vi "Dashboard Main.vi"() -> ()   [LabVIEW 2011]
uses:
  <vilib>/Rock Robotics/WPI/Camera/WPI_CameraImageSize.ctl
  <vilib>/Rock Robotics/WPI/DriverStation/WPI_DriverStationDigitalData.ctl
  <vilib>/Rock Robotics/WPI/Camera/WPI_CameraWhite Balance Values.ctl
  <vilib>/vision/NI_Vision_Development_Module.lvlib
panel:
  out "fps":dbl
  in  "Miliseconds":u32=500
  in  "Camera Settings":T2={"FPS"=10, "Compression"=30, "Image Size"=enum."320x240"}
  out "Processed Image":T3(plugin-control)
  out "Original Image":T3(plugin-control)
  in  "Annotate":bool=TRUE
  in  "Processing":enum32{"Color", "Intensity", "Intensity Open"}(tab)
  in  "Luminance":i32=255
  in  "Saturation":i32=255
  in  "Hue":i32(knob)=65 scale=0.0..255.0
  in  "Margins":cluster{"Hue":i32, "Sat":i32, "Lum":i32}={"Hue"=9, "Sat"=40, "Lum"=19} {"Sat" scale=0.0..40.0; "Lum" scale=0.0..40.0; "Hue" scale=0.0..40.0}
  in  "Range":cluster{"Lower value":sgl, "Upper value":sgl}={"Lower value"=150.0, "Upper value"=255.0} {"Lower value" scale=0.0..255.0; "Upper value" scale=0.0..255.0}
  in  "Range 2":cluster{"Lower value":sgl, "Upper value":sgl}={"Lower value"=150.0, "Upper value"=255.0} {"Lower value" scale=0.0..255.0; "Upper value" scale=0.0..255.0}
  out "Target Info":T4(array[cluster])
  in  "Particle Count Limit":i32=10
  in  "Area Size Limit":i32=444
  in  "Score Limits":T5={"Rect Coverage"=76.0, "Aspect Ratio"=70.0, "X Edge Strength"=40.0, "Y Edge Strength"=60.0}
  in  "Camera Type":enum16{"206", "1011"}(ring)
  in  "Viewer":enum32{"Camera Image", "Kinect Skeleton"}(tab)
  in  "Video Enable":bool=TRUE
  out "Camera Image":T3(plugin-control)
  out "Buttons 1":cluster{"1":bool, "2":bool, "3":bool}
  out "Kinect 1":cluster{"X":dbl, "Y":dbl, "Z":dbl} {"X" scale=1.0..-1.0; "Y" scale=1.0..-1.0; "Z" scale=1.0..-1.0}
  out "Buttons 2":cluster{"1":bool, "2":bool, "3":bool}
  out "Kinect 2":cluster{"X":dbl, "Y":dbl, "Z":dbl} {"X" scale=1.0..-1.0; "Y" scale=1.0..-1.0; "Z" scale=1.0..-1.0}
  out "Version":string
  out "Skeleton Picture":picture
  out "Players":i8
  out "Dashboard Datatype Warning":string="Warning: The Dashboard Datatype used by the robot project and this dashboard do not match.\nSee diagram for more details."
  out "Robot IP Address":string
  out "Image Error Message":string="Timeout in Camera Communications"
  # "Communications"
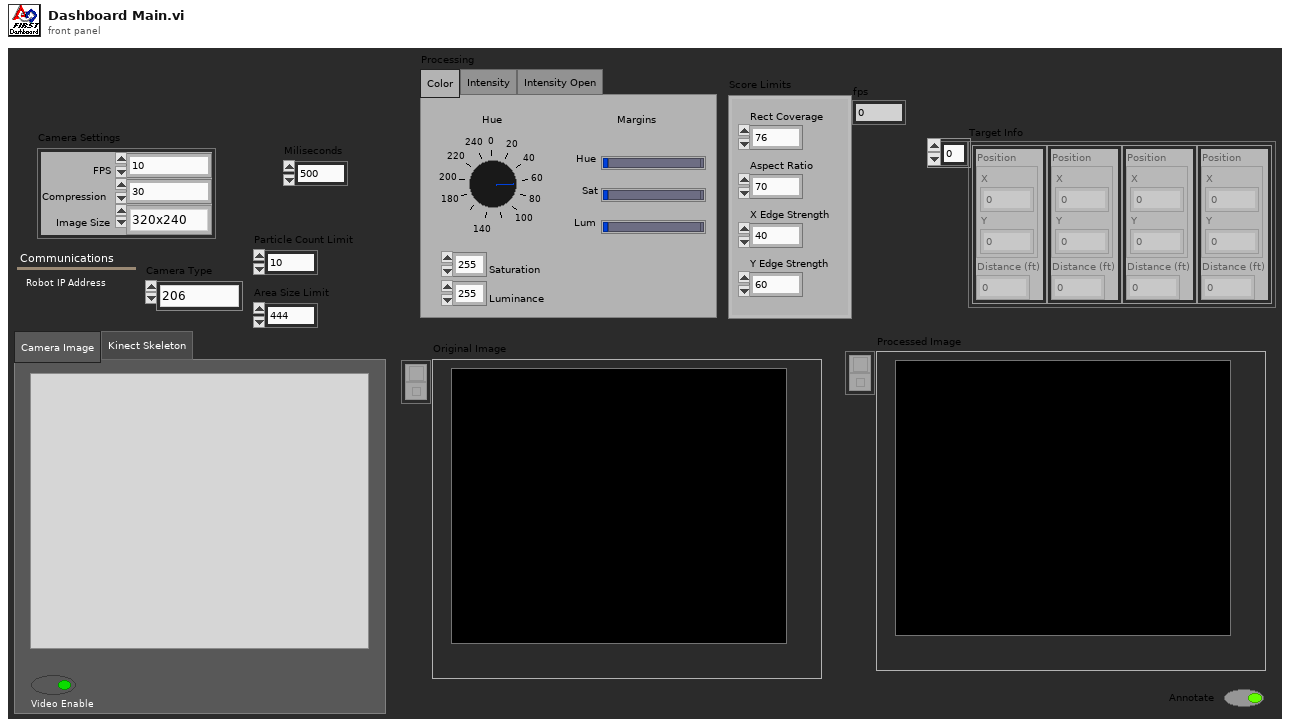
[diagram p1: front panel]
types:
  T1 = typedef "WPI_CameraImageSize.ctl" = enum16{"640x480", "320x240", "160x120"}
  T2 = cluster{"FPS":i32, "Compression":i32, "Image Size":T1}
  T3 = typedef "IMAQ Image.ctl" = refnum<image>
  T4 = cluster{"Position":cluster{"X":dbl, "Y":dbl}, "Distance (ft)":dbl}[]
  T5 = cluster{"Rect Coverage":dbl, "Aspect Ratio":dbl, "X Edge Strength":dbl, "Y Edge Strength":dbl}
  T6 = typedef "WPI_CameraWhite Balance Values.ctl" = enum16{"Auto", "Fixed indoor", "Fixed outdoor 1", "Fixed outdoor 2", "Fixed fluorescent 1", "Fixed fluorescent 2", "Hold current"}
  T7 = typedef "Image Type" = u32
  T8 = typedef "WPI_DriverStationDigitalData.ctl" = cluster{"Relay Fwd":u8, "Relay Rev":u8, "GPIO":u16, "GPIO_OE":u16, "PWM":cluster{"PWM[0]":u8, "PWM[1]":u8, "PWM[2]":u8, "PWM[3]":u8, "PWM[4]":u8, "PWM[5]":u8, "PWM[6]":u8, "PWM[7]":u8, "PWM[8]":u8, "PWM[9]":u8}}
  T9 = cluster{cluster{"AnalogModule[0]":cluster{"Channel[0]":sgl, "Channel[1]":sgl, "Channel[2]":sgl, "Channel[3]":sgl, "Channel[4]":sgl, "Channel[5]":sgl, "Channel[6]":sgl, "Channel[7]":sgl}, "AnalogModule[1]":cluster{"Channel[0]":sgl, "Channel[1]":sgl, "Channel[2]":sgl, "Channel[3]":sgl, "Channel[4]":sgl, "Channel[5]":sgl, "Channel[6]":sgl, "Channel[7]":sgl}}, cluster{"DigitalModule[0]":T8, "DigitalModule[1]":T8}, "Solenoid":u8}
  T10 = typedef "WPI_CameraDevRef.ctl" = cluster{"Camera Address":string, "CameraStatus":errorcluster, "Acquire Image Notifier":refnum<notifier>}
  T11 = typedef "LVBoundsTypeDef.ctl" = cluster{"Width":u32, "Height":u32}
  T12 = typedef "SkeletonTrackState.ctl" = enum32{"NotTracked", "PositionOnly", "Tracked"}
  T13 = cluster{"TrackingState":u8[], "Position":cluster{"x":sgl, "y":sgl, "z":sgl}, cluster{"x":sgl, "y":sgl, "z":sgl, sgl}[], "TrackState":T12}
  T14 = cluster{cluster{"ScaledToPercentRange":dbl, "ScaledToPercentRange":dbl, "ScaledToPercentRange":dbl}, cluster{bool, bool, bool}}[]
  T15 = cluster{cluster{"ScaledToPercentRange":dbl, "ScaledToPercentRange":dbl, "ScaledToPercentRange":dbl}, cluster{bool, bool, bool}}
  T16 = cluster{"ScaledToPercentRange":dbl, "ScaledToPercentRange":dbl, "ScaledToPercentRange":dbl}
  T17 = cluster{"Competition mode":bool, "Robot Link":bool, "Autonomous":bool, "Enabled":bool, "E-Stop":bool}
  T18 = cluster{"AnalogModule[0]":cluster{"Channel[0]":sgl, "Channel[1]":sgl, "Channel[2]":sgl, "Channel[3]":sgl, "Channel[4]":sgl, "Channel[5]":sgl, "Channel[6]":sgl, "Channel[7]":sgl}, "AnalogModule[1]":cluster{"Channel[0]":sgl, "Channel[1]":sgl, "Channel[2]":sgl, "Channel[3]":sgl, "Channel[4]":sgl, "Channel[5]":sgl, "Channel[6]":sgl, "Channel[7]":sgl}}
  T19 = cluster{"DigitalModule[0]":T8, "DigitalModule[1]":T8}
  T20 = cluster{"Channel[0]":sgl, "Channel[1]":sgl, "Channel[2]":sgl, "Channel[3]":sgl, "Channel[4]":sgl, "Channel[5]":sgl, "Channel[6]":sgl, "Channel[7]":sgl}[]
  T21 = cluster{"Channel[0]":sgl, "Channel[1]":sgl, "Channel[2]":sgl, "Channel[3]":sgl, "Channel[4]":sgl, "Channel[5]":sgl, "Channel[6]":sgl, "Channel[7]":sgl}
  T22 = typedef "LVRectTypeDef.ctl" = cluster{"left":i16, "top":i16, "right":i16, "bottom":i16}
  T23 = cluster{"Left":dbl, "Top":dbl, "Right":dbl, "Bottom":dbl}
  T24 = enum32{"AutoM", "Close", "Dilate", "Erode", "Gradient", "Gradient out", "Gradient in", "Hit miss", "Open", "PClose", "POpen", "Thick", "Thin"}
  T25 = cluster{cluster{"Left":dbl, "Top":dbl, "Right":dbl, "Bottom":dbl}, dbl[]}[]
  T26 = cluster{"Target Center (-1 to 1)":cluster{"X":dbl, "Y":dbl}, "Distance (ft)":dbl}
  T27 = cluster{"Target Center (-1 to 1)":cluster{"X":dbl, "Y":dbl}, "Distance (ft)":dbl}[]
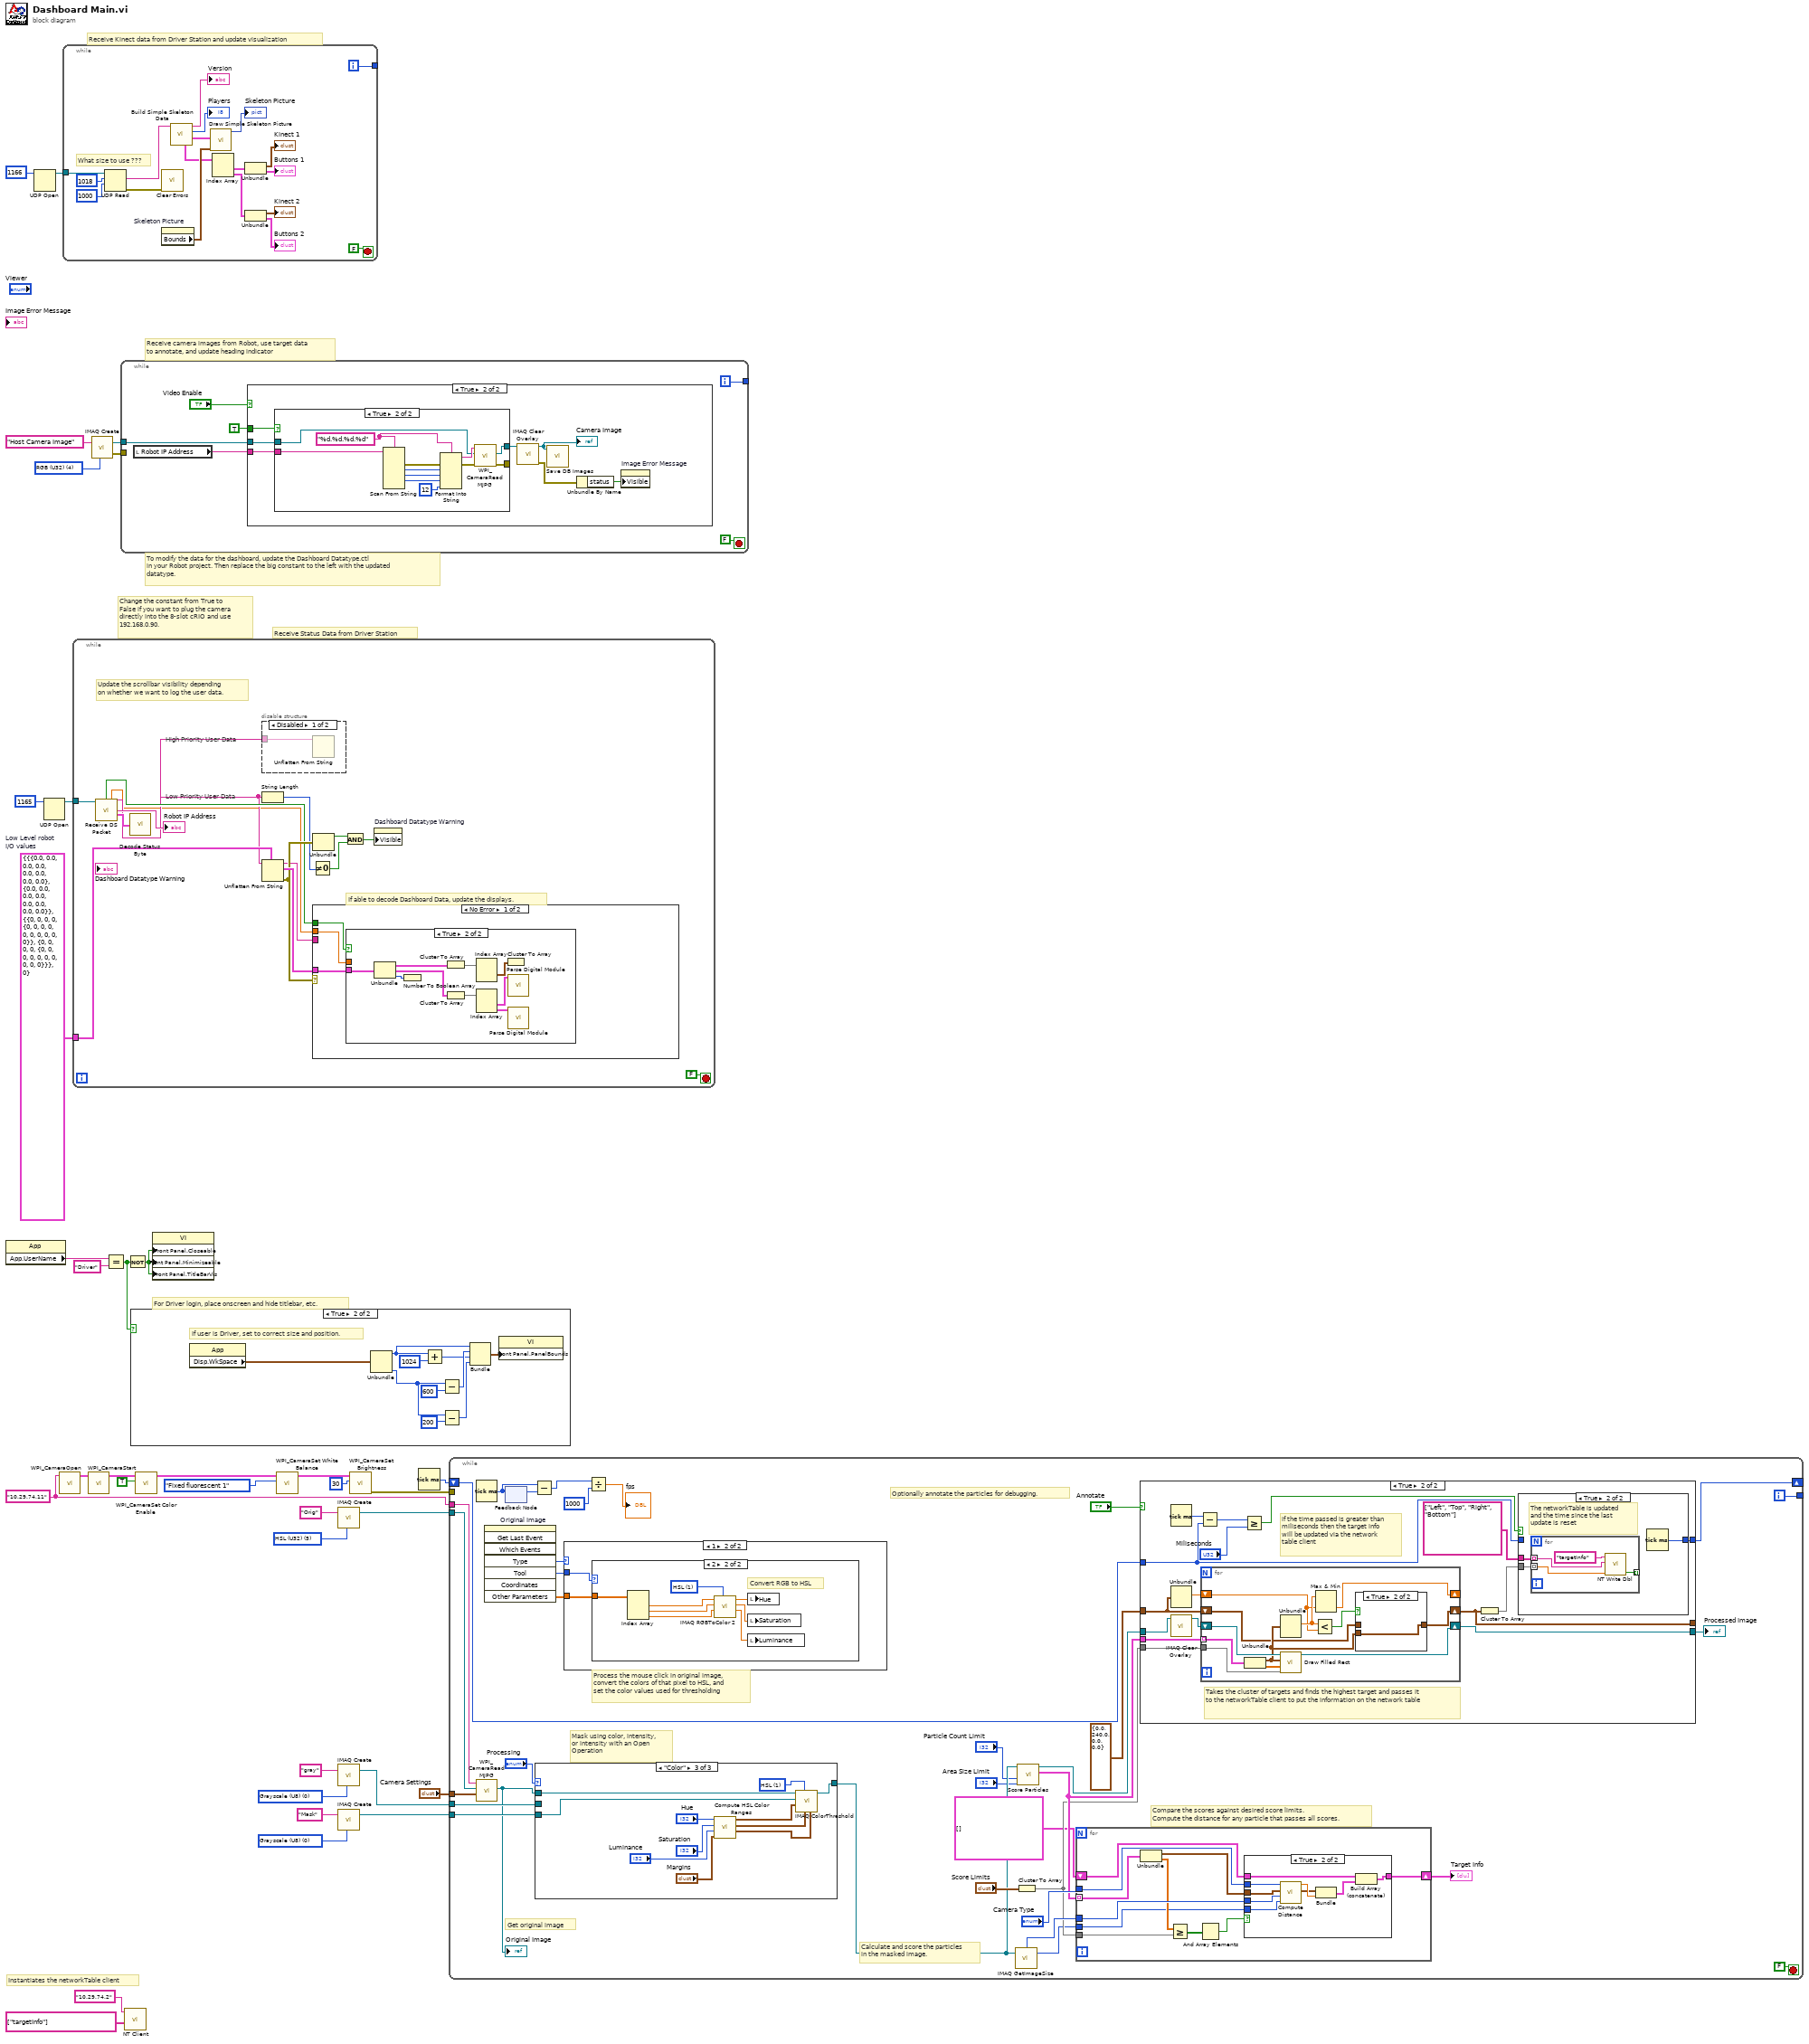
[diagram p0: block diagram]
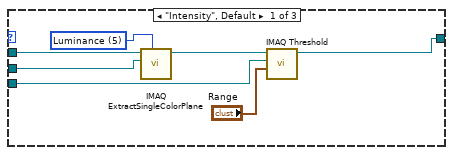
[diagram p5: hidden frame]
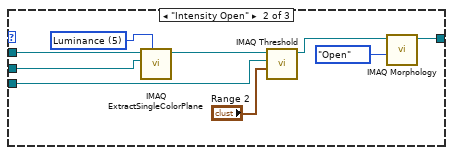
[diagram p6: hidden frame]
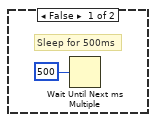
[diagram p14: hidden frame]
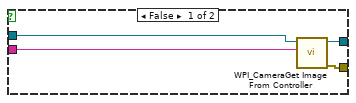
[diagram p15: hidden frame]
diagram:
  w1 = "10.29.74.11" ("Camera IP Address")
  w15 = T7 0 items=["Grayscale (U8)", "Grayscale (I16)", "Grayscale (SGL)", "Complex (CSG)", "RGB (U32)", "HSL (U32)", "RGB (U64)", "Grayscale (U16)"] ("Image Type")
  w19 = T7 5 items=["Grayscale (U8)", "Grayscale (I16)", "Grayscale (SGL)", "Complex (CSG)", "RGB (U32)", "HSL (U32)", "RGB (U64)", "Grayscale (U16)"] ("Image Type")
  w22 = T7 0 items=["Grayscale (U8)", "Grayscale (I16)", "Grayscale (SGL)", "Complex (CSG)", "RGB (U32)", "HSL (U32)", "RGB (U64)", "Grayscale (U16)"] ("Image Type")
  w25 = T9 {{"AnalogModule[0]"={"Channel[0]"=0.0, "Channel[1]"=0.0, "Channel[2]"=0.0, "Channel[3]"=0.0, "Channel[4]"=0.0, "Channel[5]"=0.0, "Channel[6]"=0.0, "Channel[7]"=0.0}, "AnalogModule[1]"={"Channel[0]"=0.0, "Channel[1]"=0.0, "Channel[2]"=0.0, "Channel[3]"=0.0, "Channel[4]"=0.0, "Channel[5]"=0.0, "Channel[6]"=0.0, "Channel[7]"=0.0}}, {"DigitalModule[0]"={"Relay Fwd"=0, "Relay Rev"=0, "GPIO"=0, "GPIO_OE"=0, "PWM"={"PWM[0]"=0, "PWM[1]"=0, "PWM[2]"=0, "PWM[3]"=0, "PWM[4]"=0, "PWM[5]"=0, "PWM[6]"=0, "PWM[7]"=0, "PWM[8]"=0, "PWM[9]"=0}}, "DigitalModule[1]"={"Relay Fwd"=0, "Relay Rev"=0, "GPIO"=0, "GPIO_OE"=0, "PWM"={"PWM[0]"=0, "PWM[1]"=0, "PWM[2]"=0, "PWM[3]"=0, "PWM[4]"=0, "PWM[5]"=0, "PWM[6]"=0, "PWM[7]"=0, "PWM[8]"=0, "PWM[9]"=0}}}, "Solenoid"=0}  # Low Level robot I/O values
  w33 = T7 4 items=["Grayscale (U8)", "Grayscale (I16)", "Grayscale (SGL)", "Complex (CSG)", "RGB (U32)", "HSL (U32)", "RGB (U64)"] ("Image Type")
  # "Instantiates the networkTable client"
  # "Change the constant from True to\nFalse if you want to plug the camera\ndirectly into the 8-slot cRIO and use\n192.168.0.90."
  # "Receive Kinect data from Driver Station and update visualization"
  # "For Driver login, place onscreen and hide titlebar, etc."
  # "To modify the data for the dashboard, update the Dashboard Datatype.ctl\nin your Robot project. Then replace the big constant to the left with the updated\ndatatype."
  # "Receive Status Data from Driver Station"
  # "Receive camera images from Robot, use target data\nto annotate, and update heading indicator"
  n1 = property class="App"() -> ("App.UserName"=w28:string)  [unwired: 2 in, 2 out]
  n2 = UDP Open(11:u16 1166 ("port")) -> (port=w23:refnum<k16>)  [unwired: 2 in, 4 out]
  n3 = UDP Open(11:u16 1165 ("port")) -> (port=w34:refnum<k16>)  [unwired: 2 in, 4 out]
  n4 = call <vilib>:"WPI_CameraOpen.vi"("Camera Address"=w1) -> ("CameraDevRef"=w3:T10)  [unwired: 9 in, 1 out]
  n5 = while {
    tunnel: w23 -> [w52]
    tunnel: [w36] -> _
    i -> [w36]
    stop <- FALSE stop-if-true
    # "What size to use ???"
    n6 = UDP Read(connection ID=w52, max size (548)=1018 ("bytes to read"), timeout ms (25000)=1000) -> (data out=w46:string, error out=w44:errorcluster)  [unwired: 1 in, 3 out]
    n7 = call <vilib>:"Clear Errors.vi"("error in (no error)"=w44) -> ()  [unwired: 6 in, 1 out]
    n8 = property on="Skeleton Picture" class="Pict"() -> ("Bounds"=w48:T11)  [unwired: 2 in, 2 out]
    n9 = call "Build Simple Skeleton Data.vi"("data out"=w46) -> ("Skeleton Data"=w47:T13, "NumPlayers"=→"Players":i8, "Version String"=→"Version":string, "Simple Joystick Info"=w43:T14)  [unwired: 6 in, 1 out]
    n10 = call "Draw Simple Skeleton Picture.vi"("Bounds"=w48, "Simple Skeleton"=w47) -> ("new picture out"=→"Skeleton Picture":picture)  [unwired: 9 in]
    n11 = Index Array(array=w43) -> (element #1=w42:T15, element #2=w41:T15)  [unwired: 2 in]
    n12 = Unbundle(w42) -> (→"Kinect 1":T16, →"Buttons 1":cluster{bool, bool, bool})
    n13 = Unbundle(w41) -> (→"Kinect 2":T16, →"Buttons 2":cluster{bool, bool, bool})
  }
  n14 = while {
    tunnel: w34 -> [w68]
    tunnel: w25 -> [w67]
    stop <- FALSE stop-if-true
    # "High Priority User Data"
    # "Low Priority User Data"
    # "Update the scrollbar visibility depending\non whether we want to log the user data."
    # "If able to decode Dashboard Data, update the displays."
    n15 = call "Receive DS Packet.vi"("Recv Socket"=w68) -> ("New Dashboard Data"=w64:bool, "Battery"=w55:sgl, "Robot IP Address"=→"Robot IP Address":string, "Status"=w69:T17, "Low Priority User Data"=w57:string, "High Priority User Data"=w56:string)  [unwired: 1 in, 8 out]
    n16 = call "Decode Status Byte.vi"("Status Byte"=w69) -> ()  [unwired: 2 out]
    n17 = disable-structure shown="Disabled" {
      disable-tunnel: w56 -> [w71 _]
      frame Disabled {
        n18 = Unflatten From String(binary string=w71) -> ()  [unwired: 2 in, 5 out]
      }
      frame Enabled {
      }
    }
    n19 = String Length(string=w57) -> (length=w59:i32)
    n20 = Unflatten From String(type=w67, binary string=w57) -> (rest of the binary string=w60:string, value=w66:T9, error out=w65:errorcluster)  [unwired: 1 in, 2 out]
    n21 = Not Equal To 0?(x=w59) -> (x != 0?=w62:bool)
    n22 = Unbundle(w65) -> ("status"=w61:bool)  [unwired: 2 out]
    n23 = case shown="No Error" w65 {
      tunnel: w66 -> [w74 _]
      tunnel: w64 -> [w73 _]
      tunnel: w60 -> [_ _]
      tunnel: w55 -> [w72 _]
      frame No Error {
        n24 = case shown="True" w73 {
          tunnel: w74 -> [_ w79]
          tunnel: w72 -> [_ _]
          frame False {
            # "Don't update if the robot hasn't sent new data"
          }
          frame True {
            n25 = Unbundle(w79) -> (w76:T18, w77:T19, "Solenoid"=w78:u8)
            n26 = Number To Boolean Array(number=w78) -> ()  [unwired: 1 out]
            n27 = Cluster To Array(cluster=w76) -> (array=w83:T20)
            n28 = Cluster To Array(cluster=w77) -> (array=w82:T8[])
            n29 = Index Array(array=w83) -> (element #1=w75:T21)  [unwired: 2 in, 1 out]
            n30 = Index Array(array=w82) -> (element #1=w81:T8, element #2=w80:T8)  [unwired: 2 in]
            n31 = Cluster To Array(cluster=w75) -> ()  [unwired: 1 out]
            n32 = call "Parse Digital Module.vi"("DigitalModule"=w81) -> ()  [unwired: 11 out]
            n33 = call "Parse Digital Module.vi"("DigitalModule"=w80) -> ()  [unwired: 11 out]
          }
        }
      }
      frame Error {
        # "Your datatypes don't match. The Dashboard Datatype.ctl in your Robot project\nand the big constant to the left of the loop need to match."
      }
    }
    n34 = And(x=w61, y=w62) -> (x .and. y?=w63:bool)
    n35 = property on="Dashboard Datatype Warning" class="Str"("Visible"=w63) -> ()  [unwired: 2 in, 2 out]
  }
  n36 = call <vilib>:"WPI_CameraStart.vi"("CameraDevRef"=w3) -> ("CameraDevRef Out"=w2:T10)  [unwired: 9 in, 1 out]
  n37 = call "IMAQ Create"("Image Name"="Host Camera Image", "Image Type"=w33) -> ("New Image"=w31:T3, "error out"=w30:errorcluster)  [unwired: 2 in, 1 out]
  n38 = Equal?(x=w28, y="Driver") -> (x = y?=w27:bool)
  n39 = while {
    tunnel: w31 -> [w87]
    tunnel: w30 -> [_]
    tunnel: [w84] -> _
    i -> [w84]
    stop <- FALSE stop-if-true
    n40 = local read "Robot IP Address"() -> (w88:string)
    n41 = case shown="True" "Video Enable" {
      tunnel: w88 -> [_ w97]
      tunnel: w87 -> [_ w96]
      tunnel: TRUE -> [_ w91]
      frame False {
        # "Sleep for 500ms"
        n42 = Wait Until Next ms Multiple(millisecond multiple=u32 500) -> ()  [unwired: 1 out]
      }
      frame True {
        n43 = case shown="True" w91 {
          tunnel: w96 -> [w100 w107]
          tunnel: [w98 w105] -> _
          tunnel: [w99 w106] -> w93
          tunnel: w97 -> [w101 w110]
          frame False {
            n44 = call <vilib>:"WPI_CameraGet Image From Controller.vi"("Controller Address"=w101, "Image"=w100) -> ("error out"=w98:errorcluster, "Image Out"=w99:T3)  [unwired: 2 in, 6 out]
          }
          frame True {
            w102 = "%d.%d.%d.%d" ("format string")
            n45 = Scan From String(format string=w102, input string=w110) -> (error out=w109:errorcluster, output 1=w111:i32, output 2=w112:i32, output 3=w113:i32)  [unwired: 2 in, 7 out]
            n46 = Format Into String(format string=w102, error in=w109, w111, w112, w113, 12 ("IP Suffix:")) -> (resulting string=w108:string, error out=w104:errorcluster)  [unwired: 1 in]
            n47 = call <vilib>:"WPI_CameraRead MJPG.vi"("error in"=w104, "Image"=w107, "address"=w108) -> ("error out"=w105:errorcluster, "Image Out"=w106:T3)  [unwired: 7 in]
          }
        }
        n48 = call "IMAQ Clear Overlay"("Image"=w93) -> ("error out"=w94:errorcluster, "Image Out"=w92:T3)  [unwired: 2 in, 7 out]
        "Camera Image" <- w92
        n49 = call "Save DB Images.vi"("Image"=w92) -> ()  [unwired: 2 in, 1 out]
        n50 = Unbundle By Name(w94) -> ("status"=w95:bool)
        n51 = property on="Image Error Message" class="Str"("Visible"=w95) -> ()  [unwired: 2 in, 2 out]
      }
    }
  }
  n52 = call "NT Client.vi"("Requested Tables"=string[] ["targetInfo"], "server IP Address"="10.29.74.2") -> ()  [unwired: 10 in]
  n53 = Not(x=w27) -> (.not. x?=w26:bool)
  n54 = case shown="True" w27 {
    frame False {
    }
    frame True {
      # "If user is Driver, set to correct size and position."
      n55 = property class="App"() -> ("Disp.WkSpace"=w123:T22)  [unwired: 2 in, 2 out]
      n56 = Unbundle(w123) -> ("left"=w118:i16, "bottom"=w114:i16)  [unwired: 2 out]
      n57 = Add(x=w118, y=1024) -> (x+y=w119:i32)
      n58 = Subtract(x=w114, y=600) -> (x-y=w120:i32)
      n59 = Subtract(x=w114, y=200) -> (x-y=w115:i32)
      n60 = Bundle("left"=w118, w120, w119, w115) -> (w122:cluster{"left":i16, i32, i32, i32})  [unwired: 1 out]
      n61 = property class="VI"("Front Panel.PanelBounds"=w122) -> ()  [unwired: 2 in, 2 out]
    }
  }
  n62 = call <vilib>:"WPI_CameraSet Color Enable.vi"("Color Enabled"=TRUE, "CameraDevRef"=w2) -> ("CameraDevRef Out"=w12:T10)  [unwired: 8 in, 1 out]
  n63 = property class="VI"("Front Panel.Closeable"=w26, "Front Panel.Minimizeable"=w26, "Front Panel.TitleBarVis"=w26) -> ()  [unwired: 2 in, 2 out]
  n64 = call <vilib>:"WPI_CameraSet White Balance.vi"("White Balance"=WPI_CameraWhite_Balance_Values."Fixed fluorescent 1", "CameraDevRef"=w12) -> ("CameraDevRef Out"=w10:T10)  [unwired: 8 in, 1 out]
  n65 = call "IMAQ Create"("Image Name"="Orig", "Image Type"=w19) -> ("New Image"=w18:T3)  [unwired: 2 in, 2 out]
  n66 = call "IMAQ Create"("Image Name"="gray", "Image Type"=w22) -> ("New Image"=w17:T3)  [unwired: 2 in, 2 out]
  n67 = call "IMAQ Create"("Image Name"="Mask", "Image Type"=w15) -> ("New Image"=w14:T3)  [unwired: 2 in, 2 out]
  n68 = call <vilib>:"WPI_CameraSet Brightness.vi"("Brightness"=30, "CameraDevRef"=w10) -> ("error out"=w8:errorcluster)  [unwired: 8 in, 1 out]
  n69 = Tick Count (ms)() -> (millisecond timer value=w4:u32)
  n70 = while {
    tunnel: w18 -> [w129]
    tunnel: w17 -> [w157]
    tunnel: w14 -> [w156]
    tunnel: w8 -> [_]
    tunnel: "Camera Settings" -> [w126]
    shift-right: [w134] -> _
    shift-left: w4 -> [w135]
    tunnel: [w133] -> _
    tunnel: w1 -> [w127]
    i -> [w133]
    stop <- FALSE stop-if-true
    # "Optionally annotate the particles for debugging."
    # "Compare the scores against desired score limits.\nCompute the distance for any particle that passes all scores."
    # "Process the mouse click in original image,\nconvert the colors of that pixel to HSL, and\nset the color values used for thresholding"
    # "Calculate and score the particles\nin the masked image."
    # "Mask using color, intensity,\nor intensity with an Open\nOperation"
    # "Get original image"
    n71 = Tick Count (ms)() -> (millisecond timer value=w131:u32)
    n72 = call <vilib>:"WPI_CameraRead MJPG.vi"("Camera Settings"=w126, "Image"=w129, "address"=w127) -> ("Image Out"=w128:T3)  [unwired: 7 in, 1 out]
    "Original Image" <- w128
    n73 = invoke on="Original Image" class="ImageControl" method="Get Last Event"() -> ("Type"=w150:i32, "Tool"=w151:i32, "Other Parameters"=w152:sgl[])  [unwired: 8 in, 5 out]
    n74 = feedback-in #1(w131) -> ()
    n75 = feedback #1() -> (w132:u32)  [unwired: 1 in]
    n76 = Subtract(x=w131, y=w132) -> (x-y=w125:u32)
    n77 = case shown="\"Color\"" "Processing" {
      tunnel: w128 -> [w205 w214 w225]
      tunnel: w157 -> [w204 w213 _]
      tunnel: w156 -> [w202 w211 w224]
      tunnel: [w200 w207 w223] -> w141
      frame "Intensity", Default {
        w199 = 5 items=["Red", "Green", "Blue", "Hue", "Saturation", "Luminance", "Value", "Intensity"] ("Color Plane")
        n78 = call "IMAQ ExtractSingleColorPlane"("Color Plane"=w199, "Image Dst"=w204, "Image Src"=w205) -> ("Image Dst Out"=w203:T3)  [unwired: 1 in, 7 out]
        n79 = call "IMAQ Threshold"("Range"="Range", "Image Dst"=w202, "Image Src"=w203) -> ("Image Dst Out"=w200:T3)  [unwired: 3 in, 5 out]
      }
      frame "Intensity Open" {
        w206 = 5 items=["Red", "Green", "Blue", "Hue", "Saturation", "Luminance", "Value", "Intensity"] ("Color Plane")
        n80 = call "IMAQ ExtractSingleColorPlane"("Color Plane"=w206, "Image Dst"=w213, "Image Src"=w214) -> ("Image Dst Out"=w212:T3)  [unwired: 1 in, 7 out]
        n81 = call "IMAQ Threshold"("Range"="Range 2", "Image Dst"=w211, "Image Src"=w212) -> ("Image Dst Out"=w208:T3)  [unwired: 3 in, 5 out]
        n82 = call "IMAQ Morphology"("Operation"=T24."Open", "Image Src"=w208) -> ("Image Dst Out"=w207:T3)  [unwired: 8 in, 1 out]
      }
      frame "Color" {
        w222 = u16 1 items=["RGB", "HSL", "HSV", "HSI"] ("Color Mode")
        n83 = call "Compute HSL Color Ranges.vi"("Margins"="Margins", "Luminance"="Luminance", "Saturation"="Saturation", "Hue"="Hue") -> ("Lum Range"=w219:cluster{i32, i32}, "Sat Range"=w220:cluster{i32, i32}, "Hue Range"=w221:cluster{i32, i32})  [unwired: 5 in]
        n84 = call "IMAQ ColorThreshold"("Blue or Luma or Val or Inten Range"=w219, "Green or Sat Range"=w220, "Color Mode"=w222, "Red or Hue Range"=w221, "Image Dst"=w224, "Image Src"=w225) -> ("Image Dst Out"=w223:T3)  [unwired: 4 in, 1 out]
      }
    }
    n85 = case shown="1" w150 {
      tunnel: w151 -> [_ w248]
      tunnel: w152 -> [_ w247]
      frame 0, Default {
      }
      frame 1 {
        n86 = case shown="2" w248 {
          tunnel: w247 -> [_ w256]
          frame Default {
          }
          frame 2 {
            w255 = u16 1 items=["RGB", "HSL", "HSV", "HSI", "CIE L*a*b*", "CIE XYZ"] ("Color Mode")
            # "Convert RGB to HSL"
            n87 = Index Array(array=w256) -> (element #1=w254:sgl, element #2=w252:sgl, element #3=w250:sgl)  [unwired: 3 in]
            n88 = call "IMAQ RGBToColor 2"("Color Mode"=w255, "Blue value"=w250, "Green value"=w252, "Red value"=w254) -> ("Blue or Luma or Val or Inten or Z or b*value"=w249:dbl, "Green or Sat or Y or a* value"=w251:dbl, "Red or Hue or X or L* value"=w253:dbl)  [unwired: 4 in, 1 out]
            n89 = local write "Hue"(w253) -> ()
            n90 = local write "Saturation"(w251) -> ()
            n91 = local write "Luminance"(w249) -> ()
          }
        }
      }
    }
    n92 = Divide(x=w125, y=1000) -> (x/y=→"fps":dbl)
    n93 = call "IMAQ GetImageSize"("Image"=w141) -> ("Y Resolution"=w137:i32, "X Resolution"=w149:i32)  [unwired: 3 in, 1 out]
    n94 = Cluster To Array(cluster="Score Limits") -> (array=w142:dbl[])
    n95 = call "Score Particles.vi"("Area Size Limit"="Area Size Limit", "Particle Count Limit"="Particle Count Limit", "Image Refnum in"=w141) -> ("Scored Particle Info"=w144:T25, "Image Refnum out"=w148:T3)  [unwired: 7 in]
    n96 = for {
      shift-right: [w235] -> w153
      shift-left: T4 [] -> [w236]
      tunnel: w149 -> [w234]
      tunnel: w144 -> [w232] mode=indexing
      tunnel: w142 -> [w227]
      tunnel: "Camera Type" -> [w231]
      tunnel: w137 -> [w226]
      n97 = Unbundle(w232) -> (w233:T23, w228:dbl[])
      n98 = Greater Or Equal?(x=w228, y=w227) -> (x >= y?=w230:bool[])
      n99 = And Array Elements(Boolean array=w230) -> (logical AND=w229:bool)
      n100 = case shown="True" w229 {
        tunnel: w236 -> [w237 w246]
        tunnel: [w237 w245] -> w235
        tunnel: w233 -> [_ w241]
        tunnel: w234 -> [_ w243]
        tunnel: w231 -> [_ w240]
        tunnel: w226 -> [_ w238]
        frame False {
        }
        frame True {
          n101 = call "Compute Distance.vi"("Y Image Resolution"=w238, "X Image Resolution"=w243, "Bounding Box"=w241, "Camera Type"=w240) -> ("Target Center (-1 to 1)"=w239:cluster{"X":dbl, "Y":dbl}, "Distance (ft)"=w242:dbl)  [unwired: 6 in]
          n102 = Bundle("Target Center (-1 to 1)"=w239, "Distance (ft)"=w242) -> (w244:T26)  [unwired: 1 in]
          n103 = Build Array (concatenate)(w246, w244) -> (w245:T27)
        }
      }
    }
    "Target Info" <- w153
    n104 = case shown="True" "Annotate" {
      tunnel: w148 -> [w160 w176]
      tunnel: [w160 w175] -> w145
      tunnel: w144 -> [_ w173]
      tunnel: w142 -> [_ w172]
      tunnel: [w159 w169] -> _
      tunnel: T23 {"Left"=0.0, "Top"=240.0, "Right"=0.0, "Bottom"=0.0} -> [w159 w171]
      tunnel: w135 -> [w158 w162]
      tunnel: [w158 w163] -> w134
      frame False {
      }
      frame True {
        # "if the time passed is greater than\nmiliseconds then the target info\nwill be updated via the network\ntable client"
        # "Takes the cluster of targets and finds the highest target and passes it\nto the networkTable client to put the information on the network table"
        n105 = Tick Count (ms)() -> (millisecond timer value=w166:u32)
        n106 = Unbundle(w171) -> ("Top"=w170:dbl)  [unwired: 3 out]
        n107 = call "IMAQ Clear Overlay"("Image"=w176) -> ("Image Out"=w174:T3)  [unwired: 2 in, 8 out]
        n108 = Subtract(x=w166, y=w162) -> (x-y=w165:u32)
        n109 = for {
          shift-right: [w195] -> w175
          shift-left: w174 -> [w196]
          tunnel: w173 -> [w194] mode=indexing
          tunnel: w172 -> [w193]
          shift-right: [w188] -> _
          shift-left: w170 -> [w186]
          shift-right: [w190] -> w169
          shift-left: w171 -> [w189]
          n110 = Unbundle(w194) -> (w191:T23, w192:dbl[])
          n111 = Unbundle(w191) -> ("Top"=w187:dbl)  [unwired: 3 out]
          n112 = call "Draw Filled Rect.vi"("Limits"=w193, "Scores"=w192, "Bounding Box"=w191, "image in"=w196) -> ("image out"=w195:T3)  [unwired: 7 in]
          n113 = Less?(x=w187, y=w186) -> (x < y?=w185:bool)
          n114 = Max & Min(x=w187, y=w186) -> (min(x,y)=w188:dbl)  [unwired: 1 out]
          n115 = case shown="True" w185 {
            tunnel: w191 -> [_ w198]
            tunnel: [w197 w198] -> w190
            tunnel: w189 -> [w197 _]
            frame False {
            }
            frame True {
            }
          }
        }
        n116 = Greater Or Equal?(x=w165, y="Miliseconds") -> (x >= y?=w161:bool)
        n117 = Cluster To Array(cluster=w169) -> (array=w167:dbl[])
        n118 = case shown="True" w161 {
          tunnel: string[] ["Left", "Top", "Right", "Bottom"] ("Requested Tables") -> [_ w180]
          tunnel: w167 -> [_ w179]
          tunnel: [w177 w178] -> w163
          tunnel: w162 -> [w177 _]
          frame False {
            # "the time since the last networkTable\nupdate will be passed through to the\nnext loop iteration"
          }
          frame True {
            # "The networkTable is updated\nand the time since the last \nupdate is reset"
            n119 = for {
              tunnel: w180 -> [w184] mode=indexing
              tunnel: w179 -> [w183] mode=indexing
              tunnel: [w181] -> _ mode=indexing
              n120 = call "NT Write Dbl.vi"("Dbl"=w183, "Field"=w184, "Table"="targetInfo") -> ("Success"=w181:bool)  [unwired: 7 in, 1 out]
            }
            n121 = Tick Count (ms)() -> (millisecond timer value=w178:u32)
          }
        }
      }
    }
    "Processed Image" <- w145
  }
